vi "Create Facility.vi"(8 "error in (no error)":errorcluster, 9 "Log File (Use default)":path, 10 "Level (error)":T1=enum."error", 11 "Name":T2) -> (0 "error out":errorcluster)   [LabVIEW 2023, in "Log.lvclass"]
uses:
  Log.lvclass
  Log_Facilities.ctl
  Log_Level.ctl
  Log_Facility.ctl
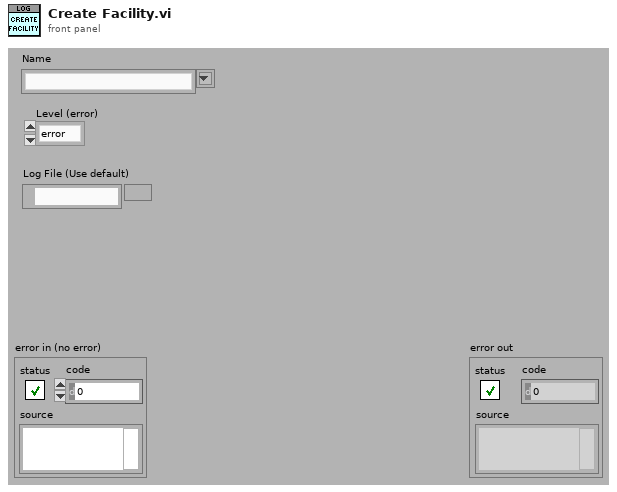
[diagram p1: front panel]
types:
  T1 = typedef "Log.lvclass/Log_Level.ctl" = enum16{"none", "info", "trace", "warn", "error", "fatal"}
  T2 = typedef "Log.lvclass/Log_Facilities.ctl" = string
  T3 = typedef "Log.lvclass/Log_Facility.ctl" = cluster{"Path":path, "Ref":refnum<file>, "Level":T1}
  T4 = enum16{"open", "replace", "create", "open or create", "replace or create", "replace or create with confirmation"}
  T5 = typedef "Log.lvclass/ObjectAttributes.ctl" = cluster{"Level":T1, "Facilities":variant, "Event":refnum<user-event>}
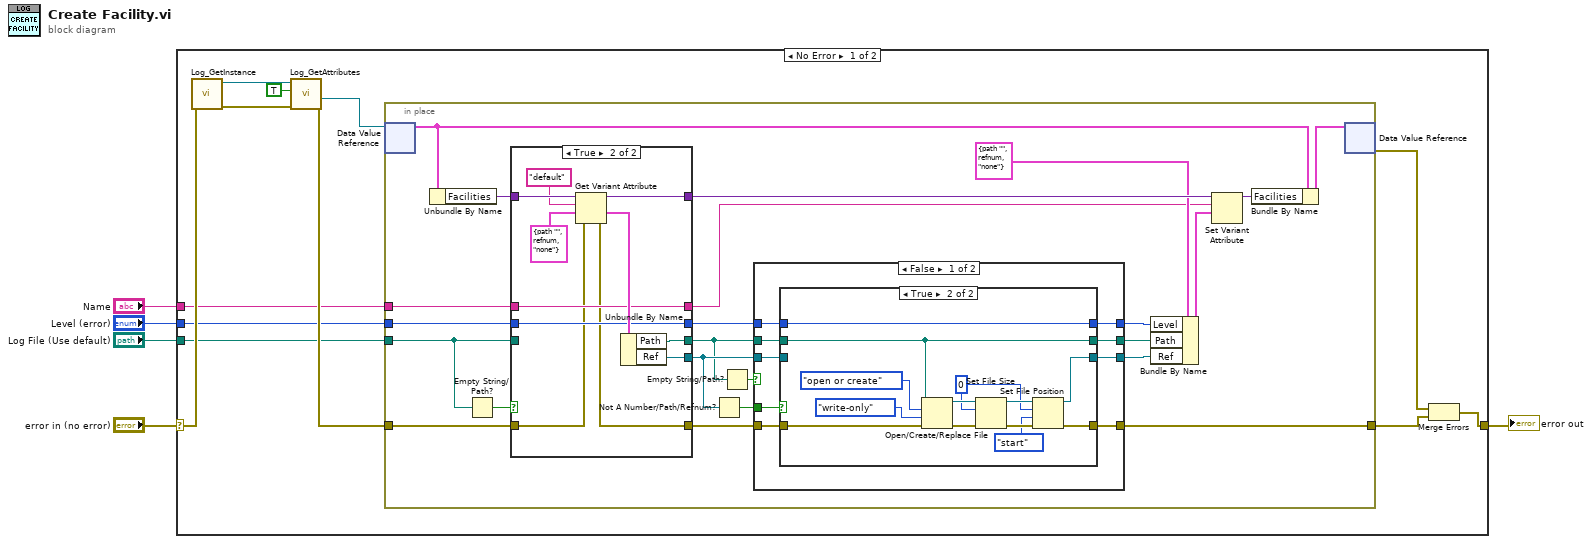
[diagram p0: block diagram]
diagram:
  n1 = case shown="No Error" "error in (no error)" {
    selector: "error in (no error)" -> [w13 w87]
    tunnel: [w16 w87] -> w4
    tunnel: "Log File (Use default)" -> [w8 _]
    tunnel: "Name" -> [w7 _]
    tunnel: "Level (error)" -> [w6 _]
    frame No Error {
      n2 = call "Log_GetInstance.vi"("error in (no error)"=w13) -> ("error out"=w15:errorcluster, "reference out"=w14:refnum<class "Log.lvclass">)  [unwired: 6 in, 3 out]
      n3 = call "Log_GetAttributes.vi"("error in (no error)"=w15, "OnlyGetDvrReference(False)"=TRUE, "reference in"=w14) -> ("error out"=w11:errorcluster, "DataRef"=w12:refnum<data-value>)  [unwired: 5 in, 2 out]
      n4 = in-place {
        in-place-border: w11 -> [w37]
        in-place-border: [w38] -> w10
        in-place-border: w8 -> [w34]
        in-place-border: w7 -> [w33]
        in-place-border: w6 -> [w32]
        n5 = in-place-dvr #1(w12) -> (w39:T5)  [unwired: 1 out]
        n6 = Unbundle By Name(w39) -> ("Facilities"=w35:variant)
        n7 = Empty String/Path?(string/path=w34) -> (empty?=w36:bool)
        n8 = case shown="True" w36 {
          tunnel: w37 -> [w71 w78]
          tunnel: w35 -> [w74 w86]
          tunnel: [w75 w82] -> w18
          tunnel: w34 -> [w75 _]
          tunnel: [w74 w81] -> w30
          tunnel: w33 -> [w72 w79]
          tunnel: w32 -> [w73 w80]
          tunnel: [w73 w80] -> w23
          tunnel: [w72 w79] -> w25
          tunnel: [w71 w77] -> w29
          tunnel: [_ w76] -> w20
          frame False {
          }
          frame True {
            n9 = Get Variant Attribute(Variant=w86, name="default", default value (empty Variant)=T3 {"Path"=path "", "Ref"=refnum, "Level"=enum."none"} ("Cluster"), error in=w78) -> (duplicate Variant=w81:variant, value=w83:T3, error out=w77:errorcluster)  [unwired: 1 out]
            n10 = Unbundle By Name(w83) -> ("Path"=w82:path, "Ref"=w76:refnum<file>)
          }
        }
        n11 = Not A Number/Path/Refnum?(number/path/refnum=w20) -> (NaN/Path/Refnum?=w24:bool)
        n12 = Empty String/Path?(string/path=w18) -> (empty?=w19:bool)
        n13 = case shown="False" w19 {
          tunnel: [w49 w67] -> w38
          tunnel: w29 -> [w48 w67]
          tunnel: [w47 w68] -> w27
          tunnel: w18 -> [w46 w69]
          tunnel: w24 -> [w45 _]
          tunnel: w23 -> [w44 w70]
          tunnel: [w43 w70] -> w22
          tunnel: [w42 w69] -> w21
          tunnel: w20 -> [w41 w68]
          frame False {
            n14 = case shown="True" w45 {
              tunnel: [w53 w58] -> w49
              tunnel: w48 -> [w53 w63]
              tunnel: [w50 w56] -> w47
              tunnel: w46 -> [w52 w61]
              tunnel: w44 -> [w51 w62]
              tunnel: [w51 w62] -> w43
              tunnel: [w52 w61] -> w42
              tunnel: w41 -> [w50 _]
              frame False {
              }
              frame True {
                w55 = i64 0 ("size (in bytes)")
                n15 = Open/Create/Replace File(file path (use dialog)=w61, error in=w63, operation (0:open)=T4."open or create", access (0:read/write)=enum16{"read/write", "read-only", "write-only"}."write-only") -> (refnum out=w59:refnum<file>, error out=w64:errorcluster)  [unwired: 2 in, 1 out]
                n16 = Set File Size(4:w64, 6:w55, 7:w59) -> (0:w60:errorcluster, 3:w57:refnum<file>)
                n17 = Set File Position(offset (in bytes) (0)=w55, refnum=w57, from (0:start)=enum16{"start", "end", "current"}."start", error in=w60) -> (refnum out=w56:refnum<file>, error out=w58:errorcluster)
              }
            }
          }
          frame True {
          }
        }
        n18 = Bundle By Name(cluster=T3 {"Path"=path "", "Ref"=refnum, "Level"=enum."none"} ("Cluster"), "Level"=w22, "Path"=w21, "Ref"=w27) -> (w26:T3)
        n19 = Set Variant Attribute(Variant=w30, name=w25, value=w26) -> (Variant out=w31:variant)  [unwired: 1 in, 2 out]
        n20 = Bundle By Name(cluster=w39, "Facilities"=w31) -> (w40:T5)
        n21 = in-place-dvr #1(w40) -> (w17:errorcluster)  [unwired: 1 out]
      }
      n22 = Merge Errors(w17, w10) -> (w16:errorcluster)
    }
    frame Error {
    }
  }
  "error out" <- w4
